vi "ExampleOnUsingFunctionalGlobalVariable.vi"() -> ()   [LabVIEW 2012]
doc: "Application example"
panel:
  out "RESISTANCE OUT":sgl format="%^_6e"
  in  "stop":bool
  # "ExampleOnUsingFunctionalGlobalVariable.vi"
  # "This is a simple example on how the continuosly and freely running AVS-47B\ncan be used in another application.  A functional global is used for \ntransferring readings  from \"FreeRunningAvs47b.vi\" to the main application.\n\nThis example starts the free-running AVS47B, but it does not have any \narrangement for stopping it. Therefore, open the block diagram, click the\nfree-running VI and stop it from its front panel."
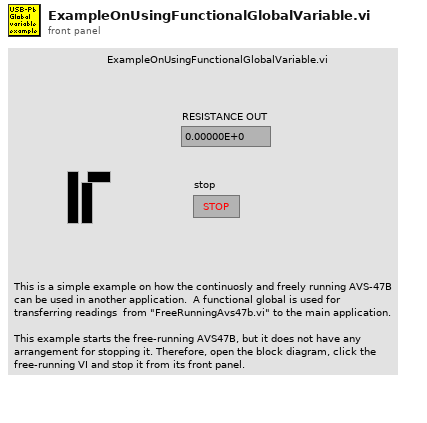
[diagram p1: front panel]
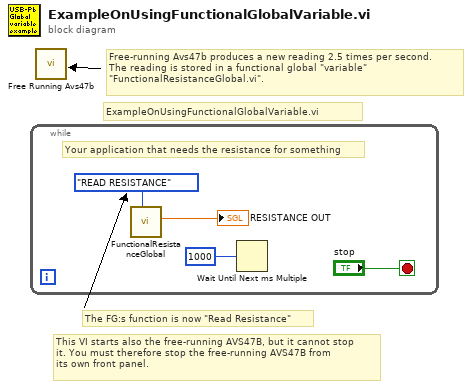
[diagram p0: block diagram]
diagram:
  # "This VI starts also the free-running AVS47B, but it cannot stop\nit. You must therefore stop the free-running AVS47B from \nits own front panel."
  # "The FG:s function is now \"Read Resistance\""
  # "ExampleOnUsingFunctionalGlobalVariable.vi"
  # "Free-running Avs47b produces a new reading 2.5 times per second.\nThe reading is stored in a functional global \"variable\"  \n\"FunctionalResistanceGlobal.vi\"."
  n1 = while {
    stop <- "stop" stop-if-true
    # "Your application that needs the resistance for something"
    n2 = call "FunctionalResistanceGlobal.vi"("FUNCTION"=enum16{"SET RESISTANCE", "READ RESISTANCE"}."READ RESISTANCE" ("FUNCTION 2")) -> ("RESISTANCE OUT"=→"RESISTANCE OUT":sgl)  [unwired: 10 in]
    n3 = Wait Until Next ms Multiple(millisecond multiple=u32 1000) -> ()  [unwired: 1 out]
  }
  n4 = call "Free Running Avs47b.vi"() -> ()  [unwired: 12 in]
